vi "Stop Publishing.vi"(8 "error in (no error)":errorcluster, 11 "Queue in":refnum<queue>) -> (0 "error out":errorcluster)   [LabVIEW 2019, in "Data Publishing Service.lvlib"]
uses:
  Data Publishing Service.lvlib
  Types/ClientType.ctl
  Types/INI Configuration.ctl
  NationalInstruments.VeriStand.ClientAPI
  <vilib>/NI VeriStand/Execution/Workspace/WorkspaceAPI.ctl
  <vilib>/NI VeriStand/Execution/Workspace/NI_VS Workspace ExecutionAPI.lvlib
  <vilib>/Skyline/Tag/Wrapper/Wrapper_class/NI Skyline Tag.lvclass
  Types/State Variables.ctl
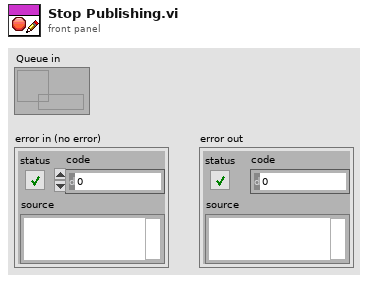
[diagram p1: front panel]
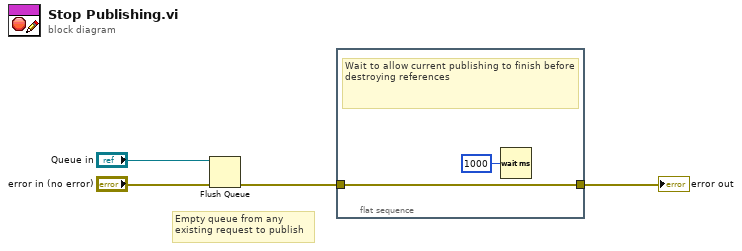
[diagram p0: block diagram]
diagram:
  # "Empty queue from any\nexisting request to publish"
  n1 = Flush Queue(queue="Queue in", error in (no error)="error in (no error)") -> (error out=w3:errorcluster)  [unwired: 2 out]
  n2 = flat-sequence {
    tunnel: [w5] -> w4
    tunnel: w3 -> [w5]
    frame #0 {
      # "Wait to allow current publishing to finish before destroying references"
      n3 = Wait (ms)(milliseconds to wait=u32 1000) -> ()  [unwired: 1 out]
    }
  }
  "error out" <- w4
